vi "ExecLog_PadString.vi"(1 "Location":enum16{"Beginnnig", "End"}(ring), 2 "Length":i32, 3 "string":string, 4 "Pad Character":string) -> (0 "String Out":string)   [LabVIEW 2017]
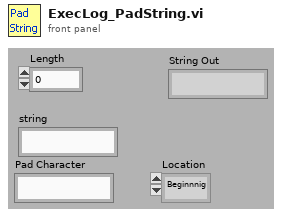
[diagram p1: front panel]
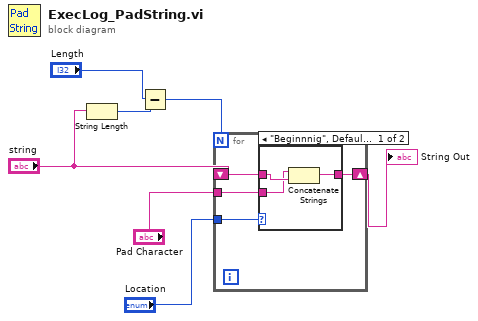
[diagram p0: block diagram]
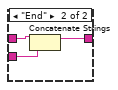
[diagram p2: hidden frame]
diagram:
  n1 = String Length(string="string") -> (length=w5:i32)
  n2 = Subtract(x="Length", y=w5) -> (x-y=w2:i32)
  n3 = for {
    N: w2 -> [_]
    shift-right: [w10] -> w7
    shift-left: "string" -> [w11]
    tunnel: "Pad Character" -> [w9]
    tunnel: "Location" -> [w8]
    n4 = case shown="\"Beginnnig\", Default" w8 {
      tunnel: w11 -> [w13 w17]
      tunnel: [w14 w16] -> w10
      tunnel: w9 -> [w12 w15]
      frame "Beginnnig", Default {
        n5 = Concatenate Strings(w12, w13) -> (w14:string)
      }
      frame "End" {
        n6 = Concatenate Strings(w17, w15) -> (w16:string)
      }
    }
  }
  "String Out" <- w7
